vi "Read From RDMA Buffer.vi"(8 "error in":errorcluster, 9 "timeout ms (25000)":i32=25000 format="%d ms", 10 "rdma session":refnum<k21>, 11 "RDMA Transceiver in":refnum<class "RDMA Transceiver.lvclass">) -> (0 "error out":errorcluster, 1 "timeout error?":bool, 2 "data":u8[](array[numeric]), 3 "RDMA Transceiver out":refnum<class "RDMA Transceiver.lvclass">)   [LabVIEW 2020, in "RDMA.lvlib" / "RDMA Transceiver.lvclass"]
doc: "Reads data from RDMA buffer."
uses:
  RDMA Transceiver.lvclass
  <vilib>/rdma/rdma.llb/RDMA Acquire Received Buffer U8.vi
  <resource>/objmgr/rdma.rc
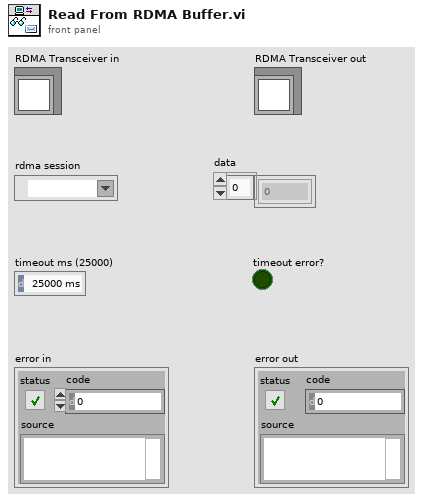
[diagram p1: front panel]
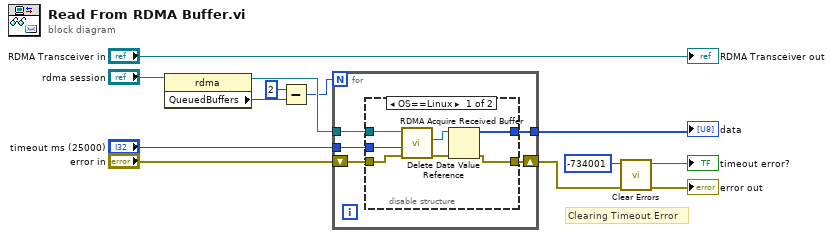
[diagram p0: block diagram]
diagram:
  # "Clearing Timeout Error"
  n1 = property class="rdma"(reference="rdma session") -> (reference out=w9:refnum<k21>, "QueuedBuffers"=w2:i64)  [unwired: 1 in, 1 out]
  n2 = Subtract(x=i64 2, y=w2) -> (x-y=w1:i64)
  n3 = for {
    N: w1 -> [_]
    tunnel: "timeout ms (25000)" -> [w18]
    tunnel: [w17] -> w10
    tunnel: w9 -> [w16]
    shift-right: [w14] -> w4
    shift-left: "error in" -> [w15]
    n4 = disable-structure shown="OS==Linux" {
      disable-tunnel: w18 -> [w25 _]
      disable-tunnel: [w23 _] -> w14
      disable-tunnel: [w22 _] -> w17
      disable-tunnel: w16 -> [w19 _]
      disable-tunnel: w15 -> [w21 _]
      frame condition #0 (active) {
        n5 = call-poly <vilib>:"RDMA Acquire Received Buffer.vi"("error in"=w21, "timeout (ms)"=w25, "rdma session in"=w19) -> ("error out"=w20:errorcluster, "edvr"=w24:refnum<data-value>)  [unwired: 6 in, 1 out]
        n6 = Delete Data Value Reference(data value reference=w24, error in=w20) -> (data value=w22:u8[], error out=w23:errorcluster)
      }
      frame condition #1 {
      }
    }
  }
  "data" <- w10
  n7 = call <vilib>:"Clear Errors.vi"("error in (no error)"=w4, "specific error code to clear (0: all)"=-734001) -> ("error out"=→"error out":errorcluster, "specific error cleared?"=→"timeout error?":bool)  [unwired: 4 in]
  "RDMA Transceiver out" <- "RDMA Transceiver in"
